vi "功能计算_何 截取位移左.vi"(0 "位移数组":dbl[](array[numeric]), 2 "拉压力数组":dbl[](array[numeric]), 3 "半行程":dbl, 5 "截取百分比":dbl) -> (14 "峰值扭矩":dbl format="%#.2f", 16 "最小扭矩":dbl, 17 "平均扭矩":dbl format="%#.2f", 19 "扭差":dbl format="%#.2f")   [LabVIEW 2013]
panel:
  out "第一个子数组":dbl[](array[numeric])
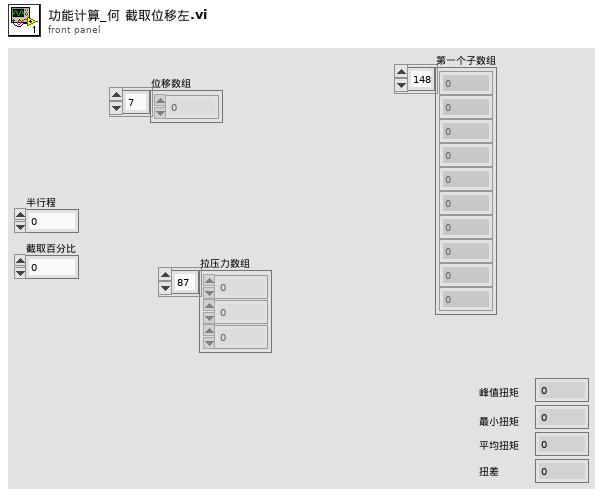
[diagram p1: front panel]
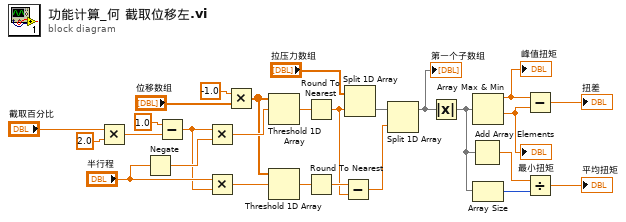
[diagram p0: block diagram]
diagram:
  n1 = Multiply(x="截取百分比", y=2.0) -> (x*y=w7:dbl)
  n2 = Negate(x="半行程") -> (-x=w11:dbl)
  n3 = Subtract(x=1.0, y=w7) -> (x-y=w10:dbl)
  n4 = Multiply(x=w10, y=w11) -> (x*y=w15:dbl)
  n5 = Multiply(x="半行程", y=w10) -> (x*y=w12:dbl)
  n6 = Multiply(x=-1.0, y="位移数组") -> (x*y=w14:dbl[])
  n7 = Threshold 1D Array(2:w15, 3:w14) -> (0:w9:dbl)  [unwired: 1 in]
  n8 = Threshold 1D Array(2:w12, 3:w14) -> (0:w8:dbl)  [unwired: 1 in]
  n9 = Round To Nearest(number=w9) -> (nearest integer value=w2:dbl)
  n10 = Round To Nearest(number=w8) -> (nearest integer value=w3:dbl)
  n11 = Subtract(x=w3, y=w2) -> (x-y=w19:dbl)
  n12 = Split 1D Array(array="拉压力数组", index=w2) -> (second subarray=w20:dbl[])  [unwired: 1 out]
  n13 = Split 1D Array(array=w20, index=w19) -> (first subarray=w24:dbl[])  [unwired: 1 out]
  "第一个子数组" <- w24
  n14 = Absolute Value(x=w24) -> (abs(x)=w26:dbl[])
  n15 = Add Array Elements(numeric array=w26) -> (sum=w27:dbl)
  n16 = Array Max & Min(array=w26) -> (max value=w23:dbl, min value=w1:dbl)  [unwired: 2 out]
  "峰值扭矩" <- w23
  "最小扭矩" <- w1
  n17 = Array Size(array=w26) -> (size(s)=w25:i32)
  n18 = Subtract(x=w23, y=w1) -> (x-y=→"扭差":dbl)
  n19 = Divide(x=w27, y=w25) -> (x/y=→"平均扭矩":dbl)
